vi "NIIE_Write INI Tokens and VI Tags.vi"(8 "Error":errorcluster, 11 "Data":T1={"Class"={"Ants"=refnum, "Layer"=refnum, "Templates"=refnum, "Icon"=refnum, "Glyph"=refnum, "Settings"=refnum, "Tools"=refnum}, "Ref"={"Add Layer"=refnum, "Remove Layer"=refnum, "Line Text"=[], "Body Text Spec"=refnum, "DNL_Font"=refnum, "glyph path str"=refnum, "templates path str"=refnum, "Arrow Up"=refnum, "Arrow Down"=refnum, "IE VI Ref"=refnum, "Glyphs tree"=refnum, "Templates tree"=refnum, "Layer Icon Text"=refnum, "Layer Template"=refnum, "Clipboard"=refnum, "BW icon in"=refnum, "Color icon in"=refnum, "Layer Clust"=refnum, "Body Text"=refnum, "DNL_Framework Templates"=refnum, "Search Templates"=refnum, "TextMarker"=refnum, "Tab Control"=refnum, "Search Glyphs"=refnum, "Line Color"=refnum, "DNL_Glyphs []"=refnum, "Fill Color"=refnum, "Tools"=refnum, "Glyphs tree"=refnum, "Icon"=refnum, "Preview"=refnum, "Ants"=refnum, "Terminals"=refnum, "menu reference"=refnum, "LayerNames"=[], "GlyphLoadAnimation"=refnum, "TemplateLoadAnimation"=refnum, "refreshGlyphs"=refnum, "refreshTemplates"=refnum}, "Support"={"AntsRect"={"left"=0, "top"=0, "right"=0, "bottom"=0}, "Mouse Move Coords"={"Horizontal"=0, "Vertical"=0}, "Mouse Down Coords"={"Horizontal"=0, "Vertical"=0}, "Temp Coord"={"Horizontal"=0, "Vertical"=0}, "Action"=enum."Default", "Edge Color"=4914962, "Fill Color"=16860, "Mouse Down?"=FALSE, "Draft Mode?"=FALSE, "Temp Icon"=bytes[3102], "CTRL Pressed"=FALSE, "Move Selection?"=FALSE, "AntsRect Orig"={"left"=0, "top"=0, "right"=0, "bottom"=0}, "Text"="", "TM Set?"=FALSE, "Mouse inside icon?"=FALSE, "Tool (old value)"=0, "Pencil Move Color"=0, "Swap Colors?"=FALSE, "Shift pressed?"=FALSE}}) -> (0 "Error Out":errorcluster, 3 "Data Out":T1={"Class"={"Ants"=refnum, "Layer"=refnum, "Templates"=refnum, "Icon"=refnum, "Glyph"=refnum, "Settings"=refnum, "Tools"=refnum}, "Ref"={"Add Layer"=refnum, "Remove Layer"=refnum, "Line Text"=[], "Body Text Spec"=refnum, "DNL_Font"=refnum, "glyph path str"=refnum, "templates path str"=refnum, "Arrow Up"=refnum, "Arrow Down"=refnum, "IE VI Ref"=refnum, "Glyphs tree"=refnum, "Templates tree"=refnum, "Layer Icon Text"=refnum, "Layer Template"=refnum, "Clipboard"=refnum, "BW icon in"=refnum, "Color icon in"=refnum, "Layer Clust"=refnum, "Body Text"=refnum, "DNL_Framework Templates"=refnum, "Search Templates"=refnum, "TextMarker"=refnum, "Tab Control"=refnum, "Search Glyphs"=refnum, "Line Color"=refnum, "DNL_Glyphs []"=refnum, "Fill Color"=refnum, "Tools"=refnum, "Glyphs tree"=refnum, "Icon"=refnum, "Preview"=refnum, "Ants"=refnum, "Terminals"=refnum, "menu reference"=refnum, "LayerNames"=[], "GlyphLoadAnimation"=refnum, "TemplateLoadAnimation"=refnum, "refreshGlyphs"=refnum, "refreshTemplates"=refnum}, "Support"={"AntsRect"={"left"=0, "top"=0, "right"=0, "bottom"=0}, "Mouse Move Coords"={"Horizontal"=0, "Vertical"=0}, "Mouse Down Coords"={"Horizontal"=0, "Vertical"=0}, "Temp Coord"={"Horizontal"=0, "Vertical"=0}, "Action"=enum."Default", "Edge Color"=4914962, "Fill Color"=16860, "Mouse Down?"=FALSE, "Draft Mode?"=FALSE, "Temp Icon"=bytes[3102], "CTRL Pressed"=FALSE, "Move Selection?"=FALSE, "AntsRect Orig"={"left"=0, "top"=0, "right"=0, "bottom"=0}, "Text"="", "TM Set?"=FALSE, "Mouse inside icon?"=FALSE, "Tool (old value)"=0, "Pencil Move Color"=0, "Swap Colors?"=FALSE, "Shift pressed?"=FALSE}})   [LabVIEW 2021]
uses:
  MB CORE/TypeDefs/Cluster_INI Data.ctl
  vi.lib/LabVIEW Icon API/lv_icon/Controls/Font.ctl
  vi.lib/LabVIEW Icon API/lv_icon/Controls/Alignment.ctl
  MB CORE/TypeDefs/Num_Font Size.ctl
  MB CORE/TypeDefs/Cluster_BodyText.ctl
  vi.lib/LabVIEW Icon API/lv_icon/Controls/IEColor.ctl
  MB CORE/TypeDefs/Cluster_Button Draw Tools.ctl
  MB CORE/TypeDefs/Bool_Draw Tool.ctl
  MB CORE/TypeDefs/Bool_Line Tool.ctl
  MB CORE/TypeDefs/Bool_ColorExtractor Tool.ctl
  MB CORE/TypeDefs/Bool_Fill Tool.ctl
  MB CORE/TypeDefs/Bool_IERect Tool.ctl
  MB CORE/TypeDefs/Bool_FRect Tool.ctl
  MB CORE/TypeDefs/Bool_Circle Tool.ctl
  MB CORE/TypeDefs/Bool_FillCircle Tool.ctl
  MB CORE/TypeDefs/Bool_Eraser Tool.ctl
  MB CORE/TypeDefs/Bool_Text Tool.ctl
  MB CORE/TypeDefs/Bool_Selection Tool.ctl
  MB CORE/TypeDefs/Bool_Move Tool.ctl
  Controls/IE Data.ctl
  Class/Ants/Ants.lvclass
  Class/FakedArray/FakedArray.lvclass
  vi.lib/LabVIEW Icon API/lv_icon/Classes/Icon/Icon.lvclass
  Class/Icon Library/Glyph.lvclass
  Class/Settings/Settings.lvclass
  Class/Tools/Tools Paint.lvclass
  Controls/IE Classes.ctl
  Controls/References Cluster.ctl
  Controls/SupportClass.ctl
  <vilib>/Utility/miscctls.llb/LVPoint32TypeDef.ctl
  Controls/ENUM_SupportClass_Action.ctl
  vi.lib/LabVIEW Icon API/lv_icon/Controls/Pathes.ctl
  vi.lib/LabVIEW Icon API/lv_icon/Controls/LabVIEW Icon Stored Information.ctl
  vi.lib/LabVIEW Icon API/lv_icon/Classes/Layer/Layer.lvclass
  vi.lib/LabVIEW Icon API/lv_icon/Classes/Icon Framework/Icon Framework.lvclass
  vi.lib/LabVIEW Icon API/lv_icon/lv_icon.lvlib
panel:
  in  "?":T8={"Show Layer Tab?"=FALSE, "Show Terminals?"=FALSE, "Text"={"Font"="", "Alignment"=0, "Size"=0}, "3rd party Templates"={"Store 3rd party Templates?"=FALSE, "Folder Name"=""}, "Merge user layers on commit"=FALSE, "Body Text"={"Line 1 text"="", "Line 2 text"="", "Line 3 text"="", "Line 4 text"="", "Line 1 color"=0, "Line 2 color"=0, "Line 3 color"=0, "Line 4 color"=0, "Body Text Spec"={"Font"="", "Alignment"=0, "Size"=3}, "Center text vertically"=FALSE, "Capitalize Text"=FALSE}, "Fill Color"=0, "Edge Color"=0, "Tab"=0, "Tool"=enum."Ellipse", "Disable Layers?"=FALSE} {"Body Text"."Body Text Spec"."Alignment" items=["left", "center", "right"]; "Text"."Alignment" items=["left", "center", "right"]}
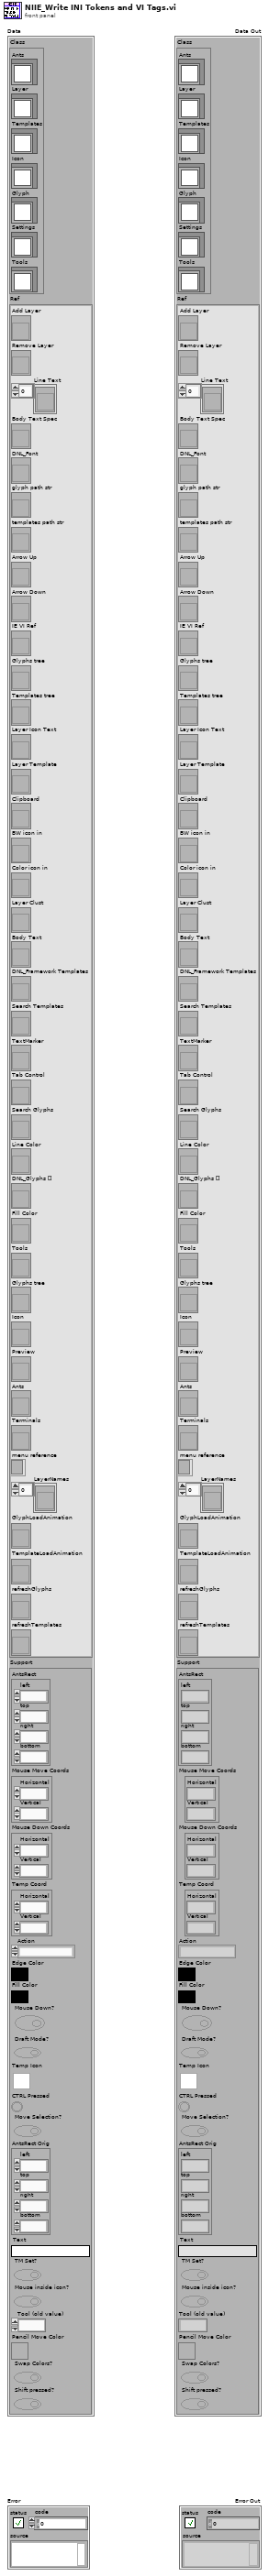
[diagram p1: front panel]
types:
  T1 = typedef "IE Data.ctl" = cluster{"Class":T2, "Ref":T3, "Support":T4}
  T2 = typedef "IE Classes.ctl" = cluster{"Ants":refnum<class "Ants.lvclass">, "Layer":refnum<class "FakedArray.lvclass">, "Templates":refnum<class "FakedArray.lvclass">, "Icon":refnum<class "Icon.lvclass">, "Glyph":refnum<class "Glyph.lvclass">, "Settings":refnum<class "Settings.lvclass">, "Tools":refnum<class "Tools Paint.lvclass">}
  T3 = typedef "References Cluster.ctl" = cluster{"Add Layer":refnum<vi>, "Remove Layer":refnum<vi>, "Line Text":refnum<vi>[], "Body Text Spec":refnum<vi>, "DNL_Font":refnum<vi>, "glyph path str":refnum<vi>, "templates path str":refnum<vi>, "Arrow Up":refnum<vi>, "Arrow Down":refnum<vi>, "IE VI Ref":refnum<vi>, "Glyphs tree":refnum<vi>, "Templates tree":refnum<vi>, "Layer Icon Text":refnum<vi>, "Layer Template":refnum<vi>, "Clipboard":refnum<vi>, "BW icon in":refnum<vi>, "Color icon in":refnum<vi>, "Layer Clust":refnum<vi>, "Body Text":refnum<vi>, "DNL_Framework Templates":refnum<vi>, "Search Templates":refnum<vi>, "TextMarker":refnum<vi>, "Tab Control":refnum<vi>, "Search Glyphs":refnum<vi>, "Line Color":refnum<vi>, "DNL_Glyphs []":refnum<vi>, "Fill Color":refnum<vi>, "Tools":refnum<vi>, "Glyphs tree":refnum<vi>, "Icon":refnum<vi>, "Preview":refnum<vi>, "Ants":refnum<vi>, "Terminals":refnum<vi>, "menu reference":refnum<k9>, "LayerNames":refnum<vi>[], "GlyphLoadAnimation":refnum<vi>, "TemplateLoadAnimation":refnum<vi>, "refreshGlyphs":refnum<vi>, "refreshTemplates":refnum<vi>}
  T4 = typedef "SupportClass.ctl" = cluster{"AntsRect":cluster{"left":i16, "top":i16, "right":i16, "bottom":i16}, "Mouse Move Coords":T5, "Mouse Down Coords":T5, "Temp Coord":T5, "Action":T6, "Edge Color":T7, "Fill Color":T7, "Mouse Down?":bool, "Draft Mode?":bool, "Temp Icon":picture, "CTRL Pressed":bool, "Move Selection?":bool, "AntsRect Orig":cluster{"left":i16, "top":i16, "right":i16, "bottom":i16}, "Text":string, "TM Set?":bool, "Mouse inside icon?":bool, "Tool (old value)":u32, "Pencil Move Color":u32, "Swap Colors?":bool, "Shift pressed?":bool}
  T5 = typedef "LVPoint32TypeDef.ctl" = cluster{"Horizontal":i32, "Vertical":i32}
  T6 = typedef "ENUM_SupportClass_Action.ctl" = enum16{"Default", "Move Selection", "Glyph Library", "Tool"}
  T7 = typedef "IEColor.ctl" = u32
  T8 = typedef "Cluster_INI Data.ctl" = cluster{"Show Layer Tab?":bool, "Show Terminals?":bool, "Text":cluster{"Font":T9, "Alignment":T10, "Size":T11}, "3rd party Templates":cluster{"Store 3rd party Templates?":bool, "Folder Name":string}, "Merge user layers on commit":bool, "Body Text":T12, "Fill Color":T7, "Edge Color":T7, "Tab":u16, "Tool":T13, "Disable Layers?":bool}
  T9 = typedef "Font.ctl" = string
  T10 = typedef "Alignment.ctl" = u16
  T11 = typedef "Num_Font Size.ctl" = u8
  T12 = typedef "Cluster_BodyText.ctl" = cluster{"Line 1 text":string, "Line 2 text":string, "Line 3 text":string, "Line 4 text":string, "Line 1 color":u32, "Line 2 color":u32, "Line 3 color":u32, "Line 4 color":u32, "Body Text Spec":cluster{"Font":T9, "Alignment":T10, "Size":u8}, "Center text vertically":bool, "Capitalize Text":bool}
  T13 = typedef "Cluster_Button Draw Tools.ctl" = enum32{"Pencil", "Line", "Dropper", "Fill", "Rectangle", "Filled Rectangle", "Ellipse", "Filled Ellipse", "Eraser", "Text", "Select", "Move"}
  T14 = enum32{"Pencil", "Line", "Dropper", "Fill", "Rectangle", "Filled Rectangle", "Ellipse", "Filled Ellipse", "Eraser", "Text", "Select", "Move"}
  T15 = cluster{"LayerIcon":picture, "LayerName":string, "Opacity":u8, "Visibility?":bool}
  T16 = enum32{"Templates", "Icon Text", "Glyphs", "Layers"}
  T17 = typedef "LabVIEW Icon Stored Information.ctl" = cluster{"Text Visible?":bool, "Text Opacity":u8, "Templ Visible?":bool, "Templ Opacity":u8, "Relative Path from 1 to 2":path, "Image":picture, "All User Layers":refnum<class "Layer.lvclass">[], "Body Text":T12}
  T18 = typedef "Pathes.ctl" = enum16{"Root Path", "Icon Templates", "Icon Templates VI", "Icon Templates Lib", "Glyphs"}
  T19 = typedef "Who Invoked Icon Editor.ctl" = cluster{"Icon Editor Invoker Type":T20, "App Refnum of Invoker":refnum<vi>, "Qualified Name of Invoker":string, "Path to Invoker":path}
  T20 = typedef "Icon Editor Invoker Type.ctl" = enum32{"Unknown Icon Source", "VI Icon", "Library Icon (any library type)", "Palette icon", "Icon from App Method"}
  T21 = typedef "Cluster_Path&Icon.ctl" = cluster{"Rectangle":cluster{"left":i16, "top":i16, "right":i16, "bottom":i16}, "Path":path, "Image":picture, "Filter":string, "FileName":string}
  T22 = cluster{"Same Folder Structure?":bool, "Folder Name":string}
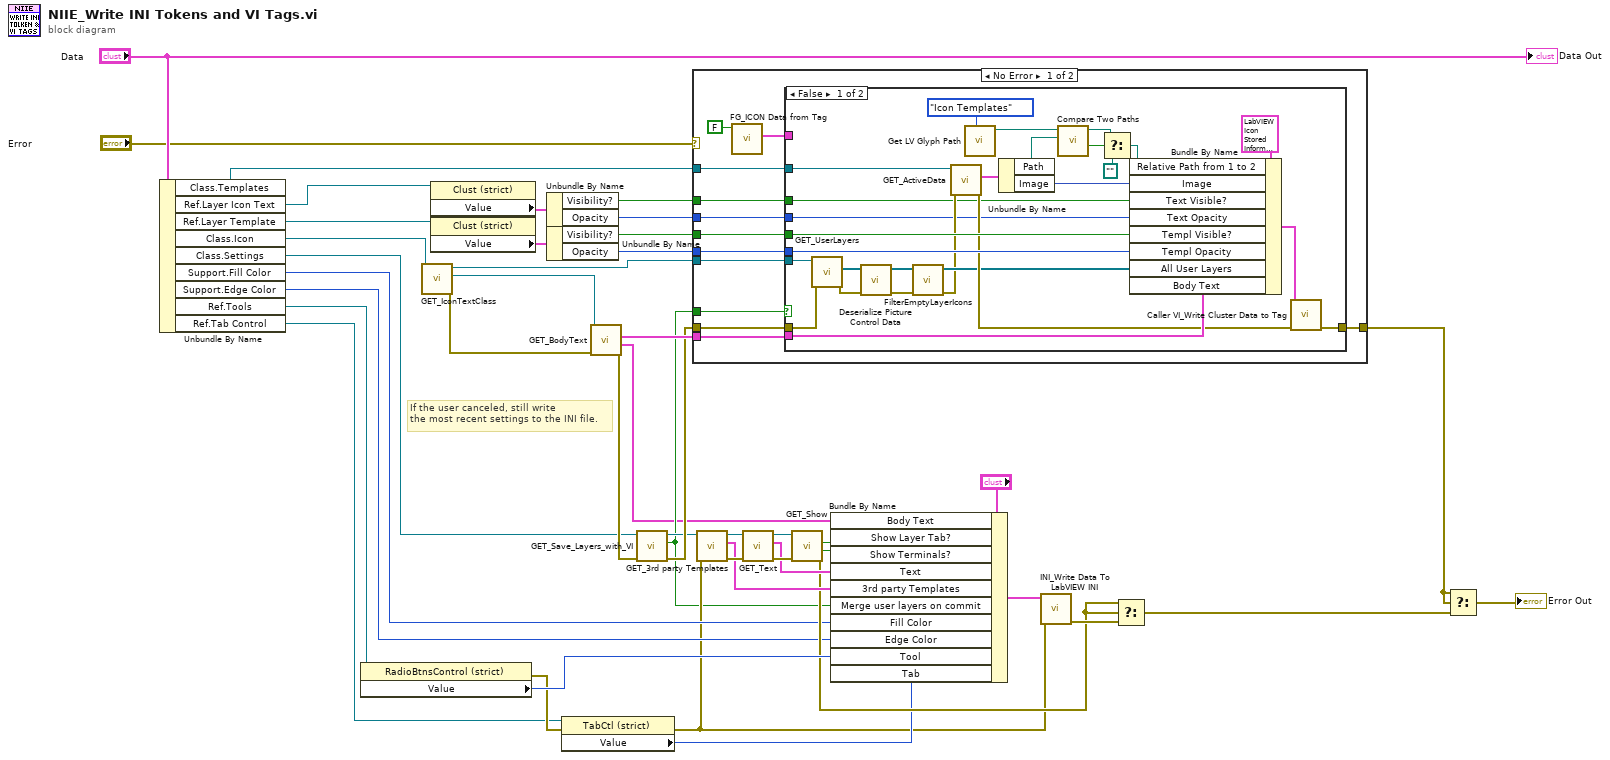
[diagram p0: block diagram]
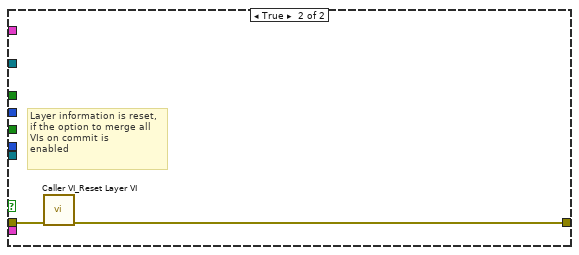
[diagram p2: hidden frame]
diagram:
  # "If the user canceled, still write\nthe most recent settings to the INI file."
  n1 = Unbundle By Name("Data") -> ("Class.Templates"=w11:refnum<class "FakedArray.lvclass">, "Ref.Layer Icon Text"=w9:refnum<vi>, "Ref.Layer Template"=w16:refnum<vi>, "Class.Icon"=w17:refnum<class "Icon.lvclass">, "Class.Settings"=w2:refnum<class "Settings.lvclass">, "Support.Fill Color"=w15:T7, "Support.Edge Color"=w14:T7, "Ref.Tools"=w13:refnum<vi>, "Ref.Tab Control"=w12:refnum<vi>)
  n2 = property class="RadioBtnsControl (strict)"(reference=w13) -> (error out=w18:errorcluster, "Value"=w27:T14)  [unwired: 1 in, 1 out]
  n3 = call-dynamic "GET_IconTextClass.vi"("Icon.lvclass in"=w17) -> ("error out"=w38:errorcluster, "Icon Framework.lvclass"=w41:refnum<class "Icon Framework.lvclass">, "Icon.lvclass out"=w40:refnum<class "Icon.lvclass">)  [unwired: 1 in, 7 out]
  n4 = property class="Clust (strict)"(reference=w9) -> ("Value"=w10:T15)  [unwired: 1 in, 2 out]
  n5 = property class="Clust (strict)"(reference=w16) -> ("Value"=w21:T15)  [unwired: 1 in, 2 out]
  n6 = Unbundle By Name(w10) -> ("Visibility?"=w7:bool, "Opacity"=w8:u8)
  n7 = Unbundle By Name(w21) -> ("Visibility?"=w19:bool, "Opacity"=w20:u8)
  n8 = property class="TabCtl (strict)"(reference=w12, error in=w18) -> (error out=w5:errorcluster, "Value"=w6:T16)  [unwired: 1 out]
  n9 = call-dynamic "GET_BodyText.vi"("error in (no error)"=w38, "Icon Framework.lvclass in"=w41) -> ("error out"=w43:errorcluster, "Cleaned Body Text"=w1:T12, "Body Text"=w39:T12)  [unwired: 7 out]
  n10 = call "GET_Save_Layers_with_VI.vi"("error in (no error)"=w43, "Settings.lvclass in"=w2) -> ("error out"=w37:errorcluster, "Merge user layers on commit"=w3:bool, "Settings.lvclass out"=w36:refnum<class "Settings.lvclass">)  [unwired: 7 out]
  n11 = case shown="No Error" "Error" {
    selector: "Error" -> [_ w87]
    tunnel: [w57 w87] -> w42
    tunnel: w40 -> [w56 _]
    tunnel: w39 -> [w55 _]
    tunnel: w37 -> [w54 _]
    tunnel: w20 -> [w53 _]
    tunnel: w19 -> [w52 _]
    tunnel: w3 -> [w51 _]
    tunnel: w11 -> [w50 _]
    tunnel: w8 -> [w49 _]
    tunnel: w7 -> [w48 _]
    frame No Error {
      n12 = call "FG_ICON Data from Tag.vi"("Init? (F)"=FALSE) -> ("Invoked Data Out"=w47:T19)  [unwired: 2 in, 8 out]
      n13 = case shown="False" w51 {
        tunnel: w56 -> [w83 _]
        tunnel: w54 -> [w79 w86]
        tunnel: w55 -> [w82 _]
        tunnel: [w78 w85] -> w57
        tunnel: w50 -> [w77 _]
        tunnel: w53 -> [w76 _]
        tunnel: w52 -> [w75 _]
        tunnel: w49 -> [w64 _]
        tunnel: w48 -> [w63 _]
        tunnel: w47 -> [_ _]
        frame False {
          n14 = call-dynamic "GET_UserLayers.vi"("error in (no error)"=w79, "Icon.lvclass in"=w83) -> ("error out"=w72:errorcluster, "All Layers"=w73:refnum<class "Layer.lvclass">[])  [unwired: 8 out]
          n15 = call "Deserialize Picture Control Data.vi"("error in (no error)"=w72, "Layers in"=w73) -> ("error out"=w66:errorcluster, "Layers out"=w68:refnum<class "Layer.lvclass">[])  [unwired: 8 out]
          n16 = call "FilterEmptyLayerIcons.vi"("error in (no error)"=w66, "Layers"=w68) -> ("error out"=w65:errorcluster, "Layers out"=w67:refnum<class "Layer.lvclass">[])  [unwired: 8 out]
          n17 = call-dynamic "GET_ActiveData.vi"("Error"=w65, "FakedArray"=w77) -> ("Error Out"=w74:errorcluster, "Path And Icon Out"=w84:T21)  [unwired: 8 out]
          n18 = call "Get LV Glyph Path.vi"("Path"=Pathes."Icon Templates") -> ("Requested Path"=w81:path)  [unwired: 2 in, 8 out]
          n19 = Unbundle By Name(w84) -> ("Path"=w80:path, "Image"=w59:picture)
          n20 = call <vilib>:"Compare Two Paths.vi"("Path 2"=w80, "Path 1"=w81) -> ("Path 2 Relative to Path 1?"=w71:bool, "Relative Path from 1 to 2"=w70:path)  [unwired: 1 in, 7 out]
          n21 = Select(t=w70, s=w71, f=path "") -> (s? t:f=w58:path)
          n22 = Bundle By Name(cluster=T17 {"Text Visible?"=FALSE, "Text Opacity"=0, "Templ Visible?"=FALSE, "Templ Opacity"=0, "Relative Path from 1 to 2"=path "", "Image"=bytes[0], "All User Layers"=[], "Body Text"={"Line 1 text"="", "Line 2 text"="", "Line 3 text"="", "Line 4 text"="", "Line 1 color"=0, "Line 2 color"=0, "Line 3 color"=0, "Line 4 color"=0, "Body Text Spec"={"Font"="", "Alignment"=0, "Size"=3}, "Center text vertically"=FALSE, "Capitalize Text"=FALSE}} ("Icon data"), "Relative Path from 1 to 2"=w58, "Image"=w59, "Text Visible?"=w63, "Text Opacity"=w64, "Templ Visible?"=w75, "Templ Opacity"=w76, "All User Layers"=w67, "Body Text"=w82) -> (w62:T17)
          n23 = call "Caller VI_Write Cluster Data to Tag.vi"("error in (no error)"=w74, "Icon data"=w62) -> ("error out"=w78:errorcluster)  [unwired: 9 in]
        }
        frame True {
          # "Layer information is reset,\nif the option to merge all \nVIs on commit is\nenabled"
          n24 = call "Caller VI_Reset Layer VI.vi"("error in (no error)"=w86) -> ("error out"=w85:errorcluster)  [unwired: 10 out]
        }
      }
    }
    frame Error {
    }
  }
  n25 = call-dynamic "GET_3rd party Templates.vi"("error in (no error)"=w5, "Settings.lvclass in"=w36) -> ("error out"=w33:errorcluster, "3rd party Templates"=w26:T22, "Settings.lvclass out"=w35:refnum<class "Settings.lvclass">)  [unwired: 7 out]
  n26 = call-dynamic "GET_Text.vi"("error in (no error)"=w33, "Settings.lvclass in"=w35) -> ("error out"=w32:errorcluster, "Text"=w25:cluster{"Font":T9, "Alignment":T10, "Size":T11}, "Settings.lvclass out"=w34:refnum<class "Settings.lvclass">)  [unwired: 7 out]
  n27 = call-dynamic "GET_Show.vi"("error in (no error)"=w32, "Settings.lvclass in"=w34) -> ("error out"=w22:errorcluster, "Show Terminals?"=w24:bool, "Show LayerTab?"=w23:bool)  [unwired: 7 out]
  n28 = Bundle By Name(cluster="?", "Body Text"=w1, "Show Layer Tab?"=w23, "Show Terminals?"=w24, "Text"=w25, "3rd party Templates"=w26, "Merge user layers on commit"=w3, "Fill Color"=w15, "Edge Color"=w14, "Tool"=w27, "Tab"=w6) -> (w31:T8)
  n29 = call "INI_Write Data To LabVIEW INI.vi"("error in (no error)"=w5, "INI Data"=w31) -> ("error out"=w28:errorcluster)  [unwired: 9 out]
  n30 = Select(t=w22, s=w22, f=w28) -> (s? t:f=w30:errorcluster)
  n31 = Select(t=w42, s=w42, f=w30) -> (s? t:f=→"Error Out":errorcluster)
  "Data Out" <- "Data"
